vi "Config - access RVHR reporting ini file.vi"(5 ".ini Controller":enum16{"Read", "Write"}(ring), 8 "error in":errorcluster, 10 "RVHR Settings":T1, 11 "Config File Ref":T2=refnum) -> (0 "error out":errorcluster, 2 "HLC Controls Out":T1, 3 "refnum out":T2)   [LabVIEW 2023]
doc: "This subVI reads initial config data from a .ini file to define the default UI.\n\nAuthor: D Keeling\nDate: 20/05/2012\nVersion: 1.0"
uses:
  <vilib>/Utility/config.llb/Config Data RefNum.ctl
  <vilib>/Utility/config.llb/NI_LVConfig.lvlib
  Controls/RVHR - Reporting Settings.ctl
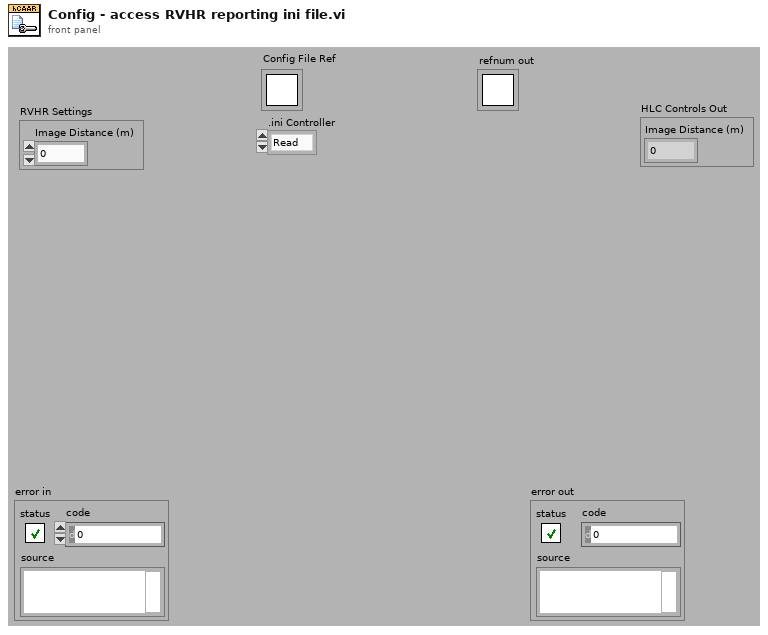
[diagram p1: front panel]
types:
  T1 = typedef "RVHR - Reporting Settings.ctl" = cluster{"Image Distance (m)":dbl}
  T2 = typedef "NI_LVConfig.lvlib/Config Data RefNum.ctl" = refnum<k1>
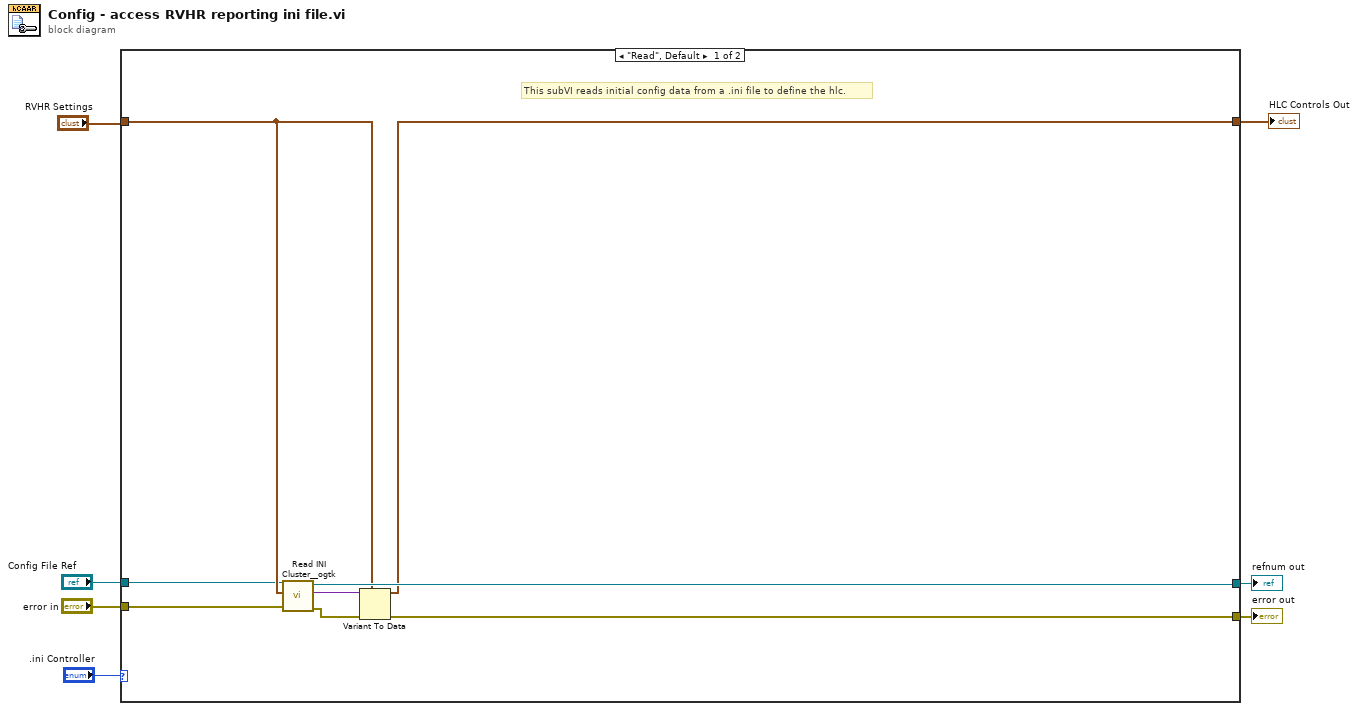
[diagram p0: block diagram]
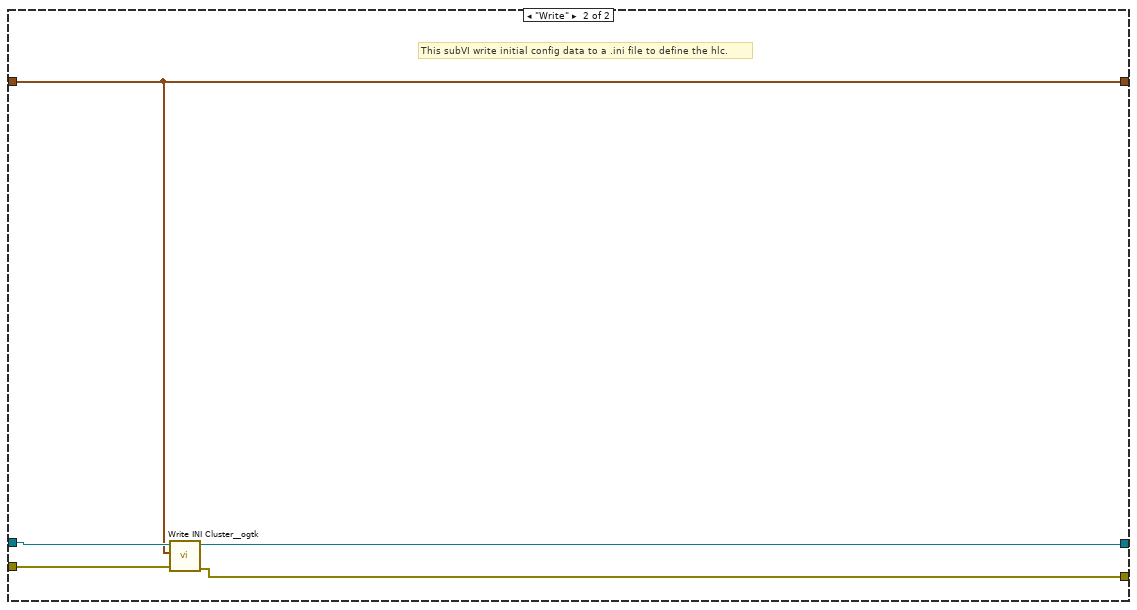
[diagram p2: hidden frame]
diagram:
  n1 = case shown="\"Read\", Default" ".ini Controller" {
    tunnel: [w14 w20] -> w6
    tunnel: "Config File Ref" -> [w8 w17]
    tunnel: [w15 w19] -> w5
    tunnel: "RVHR Settings" -> [w11 w16]
    tunnel: [w10 w16] -> w4
    tunnel: "error in" -> [w9 w18]
    frame "Read", Default {
      # "This subVI reads initial config data from a .ini file to define the hlc."
      n2 = call "Read INI Cluster__ogtk.vi"("error in (no error)"=w9, "INI Fomatted Cluster Type"=w11, "refnum"=w8) -> ("error out"=w12:errorcluster, "INI Fomatted Cluster"=w13:variant, "dup refnum"=w15:T2)  [unwired: 4 in, 2 out]
      n3 = Variant To Data(error in=w12, type=w11, Variant=w13) -> (data=w10:T1, error out=w14:errorcluster)
    }
    frame "Write" {
      # "This subVI write initial config data to a .ini file to define the hlc."
      n4 = call "Write INI Cluster__ogtk.vi"("error in (no error)"=w18, "INI Fomatted Cluster"=w16, "refnum"=w17) -> ("error out"=w20:errorcluster, "dup refnum"=w19:T2)  [unwired: 7 in]
    }
  }
  "error out" <- w6
  "refnum out" <- w5
  "HLC Controls Out" <- w4
